vi "Main_01A.vi"() -> ()   [LabVIEW 2025]
uses:
  Utility/Universal Utility/TypeDefs_Utility/Cluster_Row-Column.ctl
  9e3f57c0-2ef8-4495-8287-c6a42a5fb955.vi
  Utility/Universal Utility/TypeDefs_Utility/ENUM_4 Directions U-D-L-R.ctl
  Utility/Universal Utility/TypeDefs_Utility/ENUM_8 Directions U-D-L-R.ctl
panel:
  out "positios":i32[](array[numeric])
  out "Array 2":i32[](array[numeric])
  out "Array":bool[](array[boolean])
  out "MATCH":bool
  in  "Select Data":enum32{"Example", "Puzzle"}(tab)
  in  "Ex Answer":u32=3
  in  "Example":string="L68\nL30\nR48\nL5\nR60\nL55\nL1\nL99\nR14\nL82"
  in  "puzzel Answer":u32=1168
  in  "Puzzle":string="R46\nL11\nR26\nL29\nR14\nL26\nR18\nL38\nL48\nR45\nL8\nL48\nL2\nR34\nR4\nR8\nR35\nR41\nL16\nR31\nL36\nR16\nL22\nL35\nL33\nR42\nR42\nL43\nR28\nL31\nL38\nL47\nL29\nL13\nR13\nL17\nR16\nL20\nL16\nR18\nL21\nR41\nR37\nL10\nR48\nL44\nR26\nR17\nR7\nR78\nL90\nL33\nL91\nR74\nL56\nL53\nL90\nR97\nR42\nR30\nR17\nL47\nR4\nL4\nL23\nR23\nL66\nL45\nL82\nL23\nR90\nR70\nL29\nL66\nR51\nL54\nR54\nR32\nL48\nL95\nL57\nR63\nL14\nR86\nL67\nL45\nL39\nL35\nR19\nR19\nR45\nR87\nR89\nL83\nL57\nR22\nL22\nL36\nL53\nL95\nL616\nL87\nL13\nR67\nR933\nL70\nR75\nR74\nL16\nR20\nR17\nR45\nL92\nL64\nL61\nL28\nR541\nL42\nR1\nR27\nL77\nR850\nR39\nL39\nL373\nR66\nR53\nR16\nL28\nR66\nL7\nL68\nR355\nL80\nR52\nR48\nL16\nR13\nR78\nR330\nR995\nR57\nR643\nR31\nL26\nL1\nR96\nL93\nL48\nL59\nR..."
  out "Answer":u32
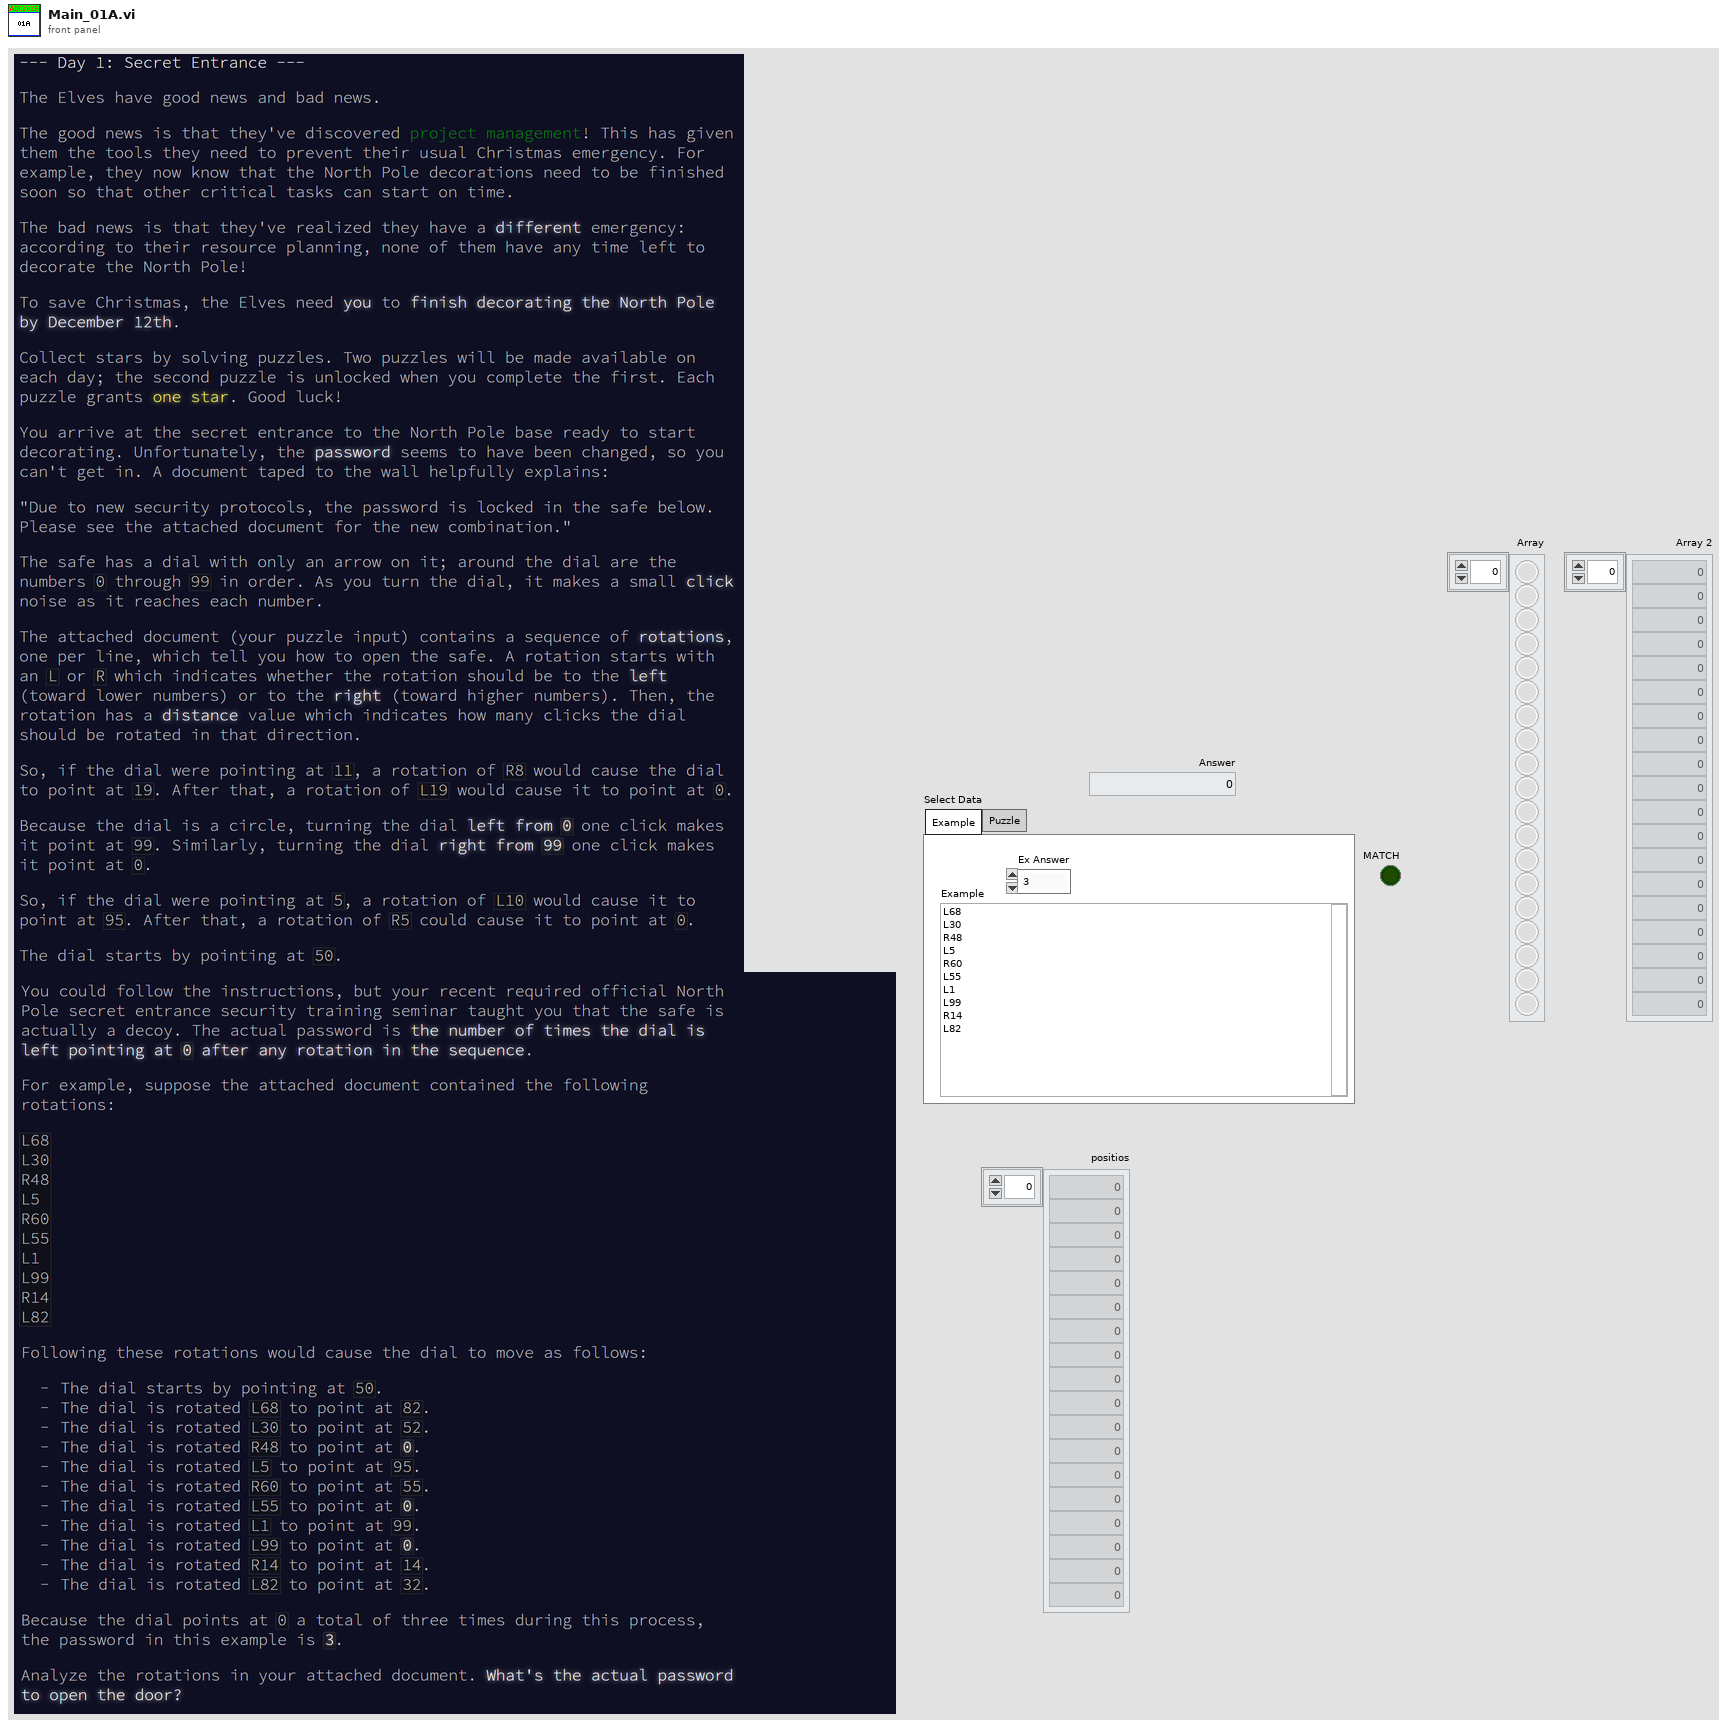
[diagram p1: front panel]
types:
  T1 = typedef "ENUM_8 Directions U-D-L-R.ctl" = enum16{"Up;-1,0", "Up-Right;-1,1", "Right;0,1", "Down-Right;1,1", "Down;1,0", "Down-Left;1,-1", "Left;0,-1", "Up-Left;-1,-1"}
  T2 = typedef "ENUM_4 Directions U-D-L-R.ctl" = enum16{"Up;-1,0", "Right;0,1", "Down;1,0", "Left;0,-1"}
  T3 = typedef "Cluster_Row-Column.ctl" = cluster{"R":i32, "C":i32}
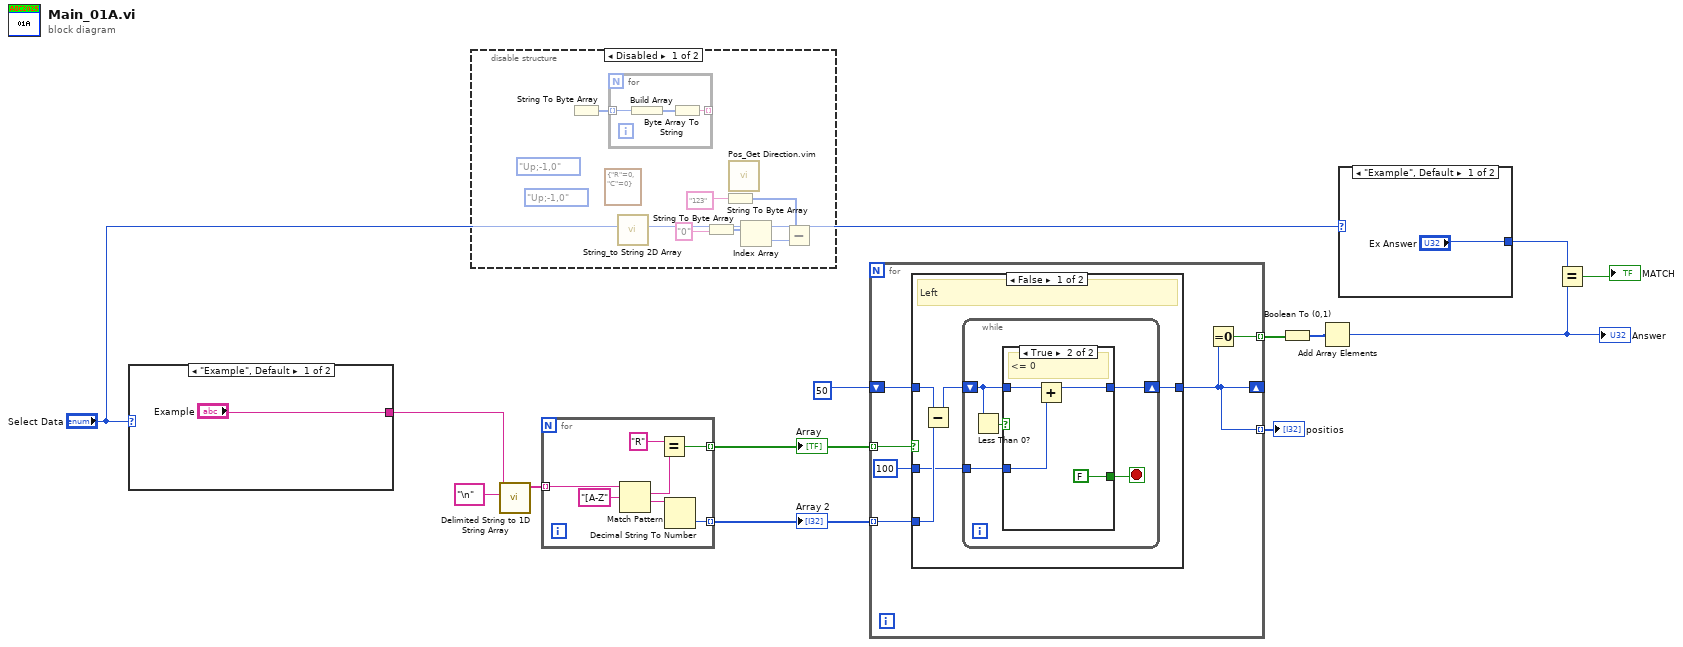
[diagram p0: block diagram]
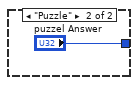
[diagram p2: hidden frame]
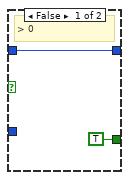
[diagram p3: hidden frame]
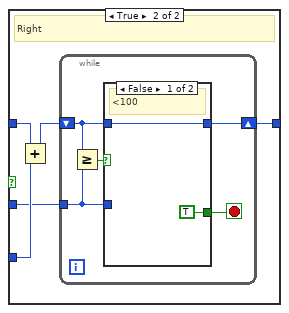
[diagram p4: hidden frame]
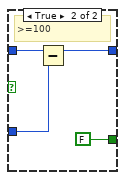
[diagram p5: hidden frame]
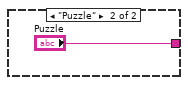
[diagram p6: hidden frame]
diagram:
  n1 = case shown="\"Example\", Default" "Select Data" {
    tunnel: ["Example" "Puzzle"] -> w11
    frame "Example", Default {
    }
    frame "Puzzle" {
    }
  }
  n2 = disable-structure shown="Disabled" {
    frame Disabled {
      (unwired) ENUM_8_Directions_U-D-L-R."Up;-1,0" ("Direction 8")
      (unwired) ENUM_4_Directions_U-D-L-R."Up;-1,0" ("Direction")
      (unwired) T3 {"R"=0, "C"=0} ("Position")
      n3 = String To Byte Array() -> (unsigned byte array=w16:u8[])  [unwired: 1 in]
      n4 = for {
        tunnel: w16 -> [w24] mode=indexing
        tunnel: [w22] -> _ mode=indexing
        n5 = Build Array(w24) -> (w23:u8[])
        n6 = Byte Array To String(unsigned byte array=w23) -> (string=w22:string)
      }
      n7 = call "String_to String 2D Array.vi"() -> ()  [unwired: 11 in, 1 out]
      n8 = String To Byte Array(string="0") -> (unsigned byte array=w19:u8[])
      n9 = String To Byte Array(string="123") -> (unsigned byte array=w17:u8[])
      n10 = call "Pos_Get Direction.vim"() -> ()  [unwired: 11 in, 1 out]
      n11 = Index Array(array=w19) -> (element=w18:u8)  [unwired: 1 in]
      n12 = Subtract(x=w17, y=w18) -> ()  [unwired: 1 out]
    }
    frame Enabled {
    }
  }
  n13 = call <vilib>:"Delimited String to 1D String Array.vi"("delimiter"="\n" ("delimiter (Tab)"), "delimited string"=w11) -> ("string array"=w12:string[])  [unwired: 9 in]
  n14 = for {
    tunnel: w12 -> [w31] mode=indexing
    tunnel: [w27] -> w9 mode=indexing
    tunnel: [w25] -> w8 mode=indexing
    n15 = Match Pattern(string=w31, regular expression="[A-Z") -> (match substring=w29:string, after substring=w26:string)  [unwired: 1 in, 2 out]
    n16 = Equal?(x="R", y=w29) -> (x = y?=w27:bool)
    n17 = Decimal String To Number(string=w26) -> (number=w25:i32)  [unwired: 2 in, 1 out]
  }
  "Array" <- w9
  "Array 2" <- w8
  n18 = for {
    shift-right: [w32] -> _
    shift-left: 50 -> [w36]
    tunnel: w9 -> [w37] mode=indexing
    tunnel: w8 -> [w35] mode=indexing
    tunnel: [w33] -> w6 mode=indexing
    tunnel: [w32] -> w7 mode=indexing
    n19 = case shown="False" w37 {
      tunnel: w36 -> [w42 w58]
      tunnel: w35 -> [w41 w57]
      tunnel: [w39 w55] -> w32
      tunnel: 100 ("y") -> [w40 w56]
      frame False {
        # "Left"
        n20 = Subtract(x=w42, y=w41) -> (x-y=w38:i32)
        n21 = while {
          tunnel: w40 -> [w46]
          shift-right: [w45] -> w39
          shift-left: w38 -> [w44]
          stop <- w43 stop-if-true
          n22 = Less Than 0?(x=w44) -> (x < 0?=w47:bool)
          n23 = case shown="True" w47 {
            tunnel: w44 -> [w48 w53]
            tunnel: w46 -> [_ w51]
            tunnel: [w48 w52] -> w45
            tunnel: [TRUE FALSE] -> w43
            frame False {
              # "> 0"
            }
            frame True {
              # "<= 0"
              n24 = Add(x=w53, y=w51) -> (x+y=w52:i32)
            }
          }
        }
      }
      frame True {
        # "Right"
        n25 = Add(x=w58, y=w57) -> (x+y=w54:i32)
        n26 = while {
          tunnel: w56 -> [w59]
          shift-right: [w62] -> w55
          shift-left: w54 -> [w61]
          stop <- w60 stop-if-true
          n27 = Greater Or Equal?(x=w61, y=w59) -> (x >= y?=w63:bool)
          n28 = case shown="False" w63 {
            tunnel: w61 -> [w64 w69]
            tunnel: w59 -> [_ w67]
            tunnel: [w64 w68] -> w62
            tunnel: [TRUE FALSE] -> w60
            frame False {
              # "<100"
            }
            frame True {
              # ">=100"
              n29 = Subtract(x=w69, y=w67) -> (x-y=w68:i32)
            }
          }
        }
      }
    }
    n30 = Equal To 0?(x=w32) -> (x = 0?=w33:bool)
  }
  "positios" <- w7
  n31 = Boolean To (0,1)(Boolean=w6) -> (0, 1=w5:i16[])
  n32 = Add Array Elements(numeric array=w5) -> (sum=w2:i16)
  "Answer" <- w2
  n33 = case shown="\"Example\", Default" "Select Data" {
    tunnel: ["Ex Answer" "puzzel Answer"] -> w3
    frame "Example", Default {
    }
    frame "Puzzle" {
    }
  }
  n34 = Equal?(x=w3, y=w2) -> (x = y?=→"MATCH":bool)
